vi "is-log-file-open.vi"(11 "Byte Stream File in":refnum<file>) -> (0 "Log File Open":bool)   [LabVIEW 2024]
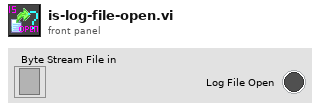
[diagram p1: front panel]
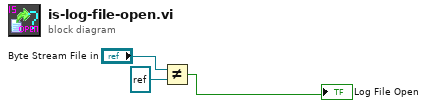
[diagram p0: block diagram]
diagram:
  n1 = Not Equal?(x="Byte Stream File in", y=refnum<file> refnum ("Byte Stream File out")) -> (x != y?=→"Log File Open":bool)
